vi "WSVCAP SHL FPGA LL I2C Read ACK.vi"(11 "error in (no error)":errorcluster, 13 "Socket Mask":u32 format="%08x") -> (4 "Long Word Out (1-Bit for Each Channel)":u32, 15 "error out":errorcluster)   [LabVIEW 2017]
uses:
  <vilib>/eio/EIONode/EIONode.xnode
  WSVCAP SHL FPGA LL I2C Debug Global.vi
  <vilib>/rvi/eio/common/nirviEmuTemplateMethod_errors.vi
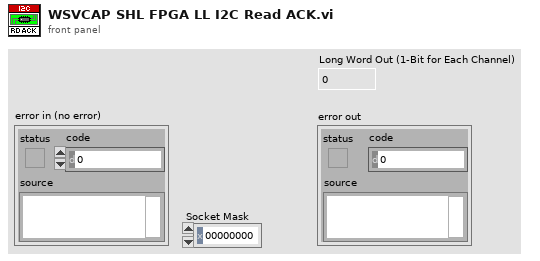
[diagram p1: front panel]
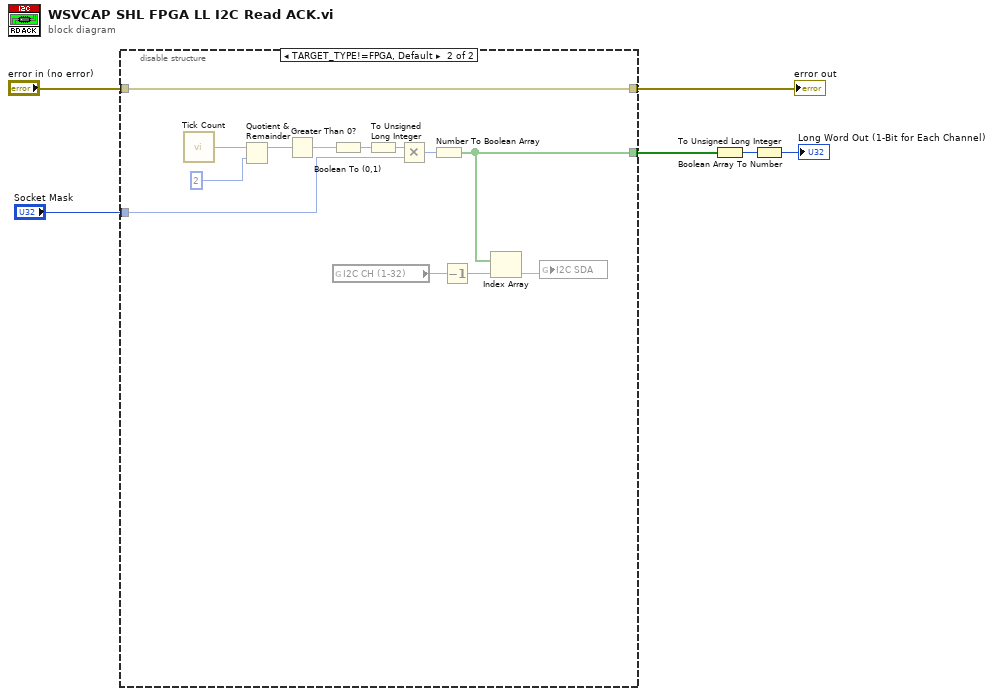
[diagram p0: block diagram]
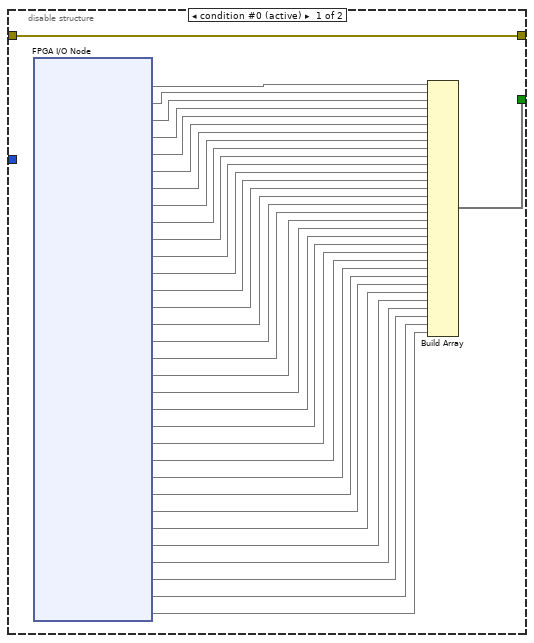
[diagram p2: hidden frame]
diagram:
  n1 = disable-structure shown="TARGET_TYPE!=FPGA, Default" {
    disable-tunnel: [w39 w44] -> w6
    disable-tunnel: [w7 w50] -> w3
    disable-tunnel: "error in (no error)" -> [w7 w50]
    disable-tunnel: "Socket Mask" -> [_ w47]
    frame condition #0 (active) {
      n2 = xnode "FPGA I/O Node"() -> ("I2C_SDAA_S1"=w40, "I2C_SDAA_S2"=w38, "I2C_SDAA_S3"=w37, "I2C_SDAA_S4"=w36, "I2C_SDAA_S5"=w35, "I2C_SDAA_S6"=w34, "I2C_SDAA_S7"=w33, "I2C_SDAA_S8"=w32, "I2C_SDAA_S9"=w31, "I2C_SDAA_S10"=w30, "I2C_SDAA_S11"=w29, "I2C_SDAA_S12"=w28, "I2C_SDAA_S13"=w27, "I2C_SDAA_S14"=w26, "I2C_SDAA_S15"=w25, "I2C_SDAA_S16"=w24, "I2C_SDAB_S1"=w23, "I2C_SDAB_S2"=w22, "I2C_SDAB_S3"=w21, "I2C_SDAB_S4"=w20, "I2C_SDAB_S5"=w19, "I2C_SDAB_S6"=w18, "I2C_SDAB_S7"=w17, "I2C_SDAB_S8"=w16, "I2C_SDAB_S9"=w15, "I2C_SDAB_S10"=w14, "I2C_SDAB_S11"=w13, "I2C_SDAB_S12"=w12, "I2C_SDAB_S13"=w11, "I2C_SDAB_S14"=w10, "I2C_SDAB_S15"=w9, "I2C_SDAB_S16"=w8)  [unwired: 32 in, 32 out]
      n3 = Build Array(w40, w38, w37, w36, w35, w34, w33, w32, w31, w30, w29, w28, w27, w26, w25, w24, w23, w22, w21, w20, w19, w18, w17, w16, w15, w14, w13, w12, w11, w10, w9, w8) -> (w39:void[])
    }
    frame condition #1 {
      n4 = call "Tick Count"() -> ("Tick Count(Ticks)"=w53:u32)
      n5 = Quotient & Remainder(x=w53, y=u32 2) -> (x-y*floor(x/y)=w52:u32)  [unwired: 1 out]
      n6 = Greater Than 0?(x=w52) -> (x > 0?=w49:bool)
      n7 = Boolean To (0,1)(Boolean=w49) -> (0, 1=w48:i16)
      n8 = global read "WSVCAP SHL FPGA LL I2C Debug Global.vi" "I2C CH (1-32)"() -> (w42:i32)
      n9 = To Unsigned Long Integer(number=w48) -> (unsigned 32bit integer=w46:u32)
      n10 = Multiply(x=w46, y=w47) -> (x*y=w45:u32)
      n11 = Number To Boolean Array(number=w45) -> (Boolean array=w44:bool[])
      n12 = Decrement(x=w42) -> (x-1=w41:i32)
      n13 = Index Array(array=w44, index=w41) -> (element=w43:bool)
      n14 = global write "WSVCAP SHL FPGA LL I2C Debug Global.vi" "I2C SDA"(w43) -> ()
    }
  }
  "error out" <- w3
  n15 = Boolean Array To Number(Boolean array=w6) -> (number=w5:u32)
  n16 = To Unsigned Long Integer(number=w5) -> (unsigned 32bit integer=→"Long Word Out (1-Bit for Each Channel)":u32)
